vi "xmlUserCheck.vi"(8 "PSW":string, 11 "Name":string) -> (2 "check passed?":bool)   [LabVIEW 2011]
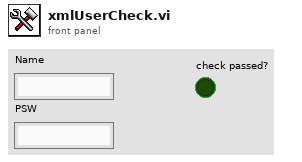
[diagram p1: front panel]
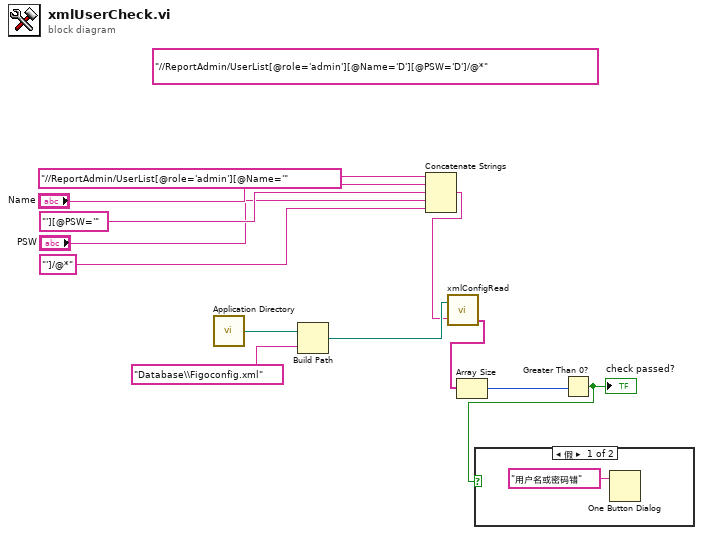
[diagram p0: block diagram]
diagram:
  (unwired) "//ReportAdmin/UserList[@role='admin'][@Name='D'][@PSW='D']/@*" ("XPath expression")
  n1 = call <vilib>:"Application Directory.vi"() -> ("Application Directory"=w12:path)
  n2 = Build Path(base path=w12, name or relative path="Database\\Figoconfig.xml" ("名称或相对路径")) -> (appended path=w10:path)
  n3 = Concatenate Strings("//ReportAdmin/UserList[@role='admin'][@Name='" ("字符串"), "Name", "'][@PSW='" ("字符串"), "PSW", "']/@*" ("字符串")) -> (w3:string)
  n4 = call "xmlConfigRead.vi"("path to XML document"=w10, "XPath expression"=w3) -> ("OutParaArray"=w9:string[])  [unwired: 2 out]
  n5 = Array Size(array=w9) -> (size(s)=w2:i32)
  n6 = Greater Than 0?(x=w2) -> (x > 0?=w1:bool)
  "check passed?" <- w1
  n7 = case shown="假" w1 {
    frame False {
      n8 = One Button Dialog(message="用户名或密码错" ("消息")) -> ()  [unwired: 1 in, 1 out]
    }
    frame True {
    }
  }
